vi "Configure Session.vi"(8 "error in":errorcluster, 11 "Plugin in":refnum<class "Dynamic Channel.lvclass">) -> (0 "error out":errorcluster, 3 "Plugin out":refnum<class "Dynamic Channel.lvclass">)   [LabVIEW 2020, in "Dynamic Channel.lvlib" / "Dynamic Channel.lvclass"]
uses:
  Dynamic Channel.lvclass
  C:/Program Files/National Instruments/LabVIEW 2020/vi.lib/FlexLogger/SDK/PluginSDK.lvlibp/PEFClasses/SDK/Plugin/Plugin.lvclass
  Dynamic Channel.lvclass/Dynamic Channel.ctl
  <vilib>/FlexLogger/SDK/PluginSDK.lvlibp/PEFClasses/SDK/Producer Channel/Producer Channel.lvclass
  C:/Program Files/National Instruments/LabVIEW 2020/vi.lib/FlexLogger/SDK/PluginSDK.lvlibp/PEFClasses/SDK/Channel/Channel.lvclass
  <vilib>/FlexLogger/SDK/PluginSDK.lvlibp/PEFClasses/SDK/Plugin/ParameterAccess/Read I32.vi
  <vilib>/FlexLogger/SDK/PluginSDK.lvlibp/PEFClasses/SDK/Plugin/ParameterAccess/Write I32.vi
  <vilib>/FlexLogger/SDK/PluginSDK.lvlibp/PEFClasses/SDK/Producer Channel/Create Producer Channel.vi
  <vilib>/FlexLogger/SDK/PluginSDK.lvlibp/PEFClasses/SDK/Channel/ParameterAccess/Write DBL.vi
  <vilib>/FlexLogger/SDK/PluginSDK.lvlibp/PEFClasses/SDK/Channel/ParameterAccess/Write Single Channel.vi
  <vilib>/FlexLogger/SDK/PluginSDK.lvlibp/PEFClasses/SDK/Plugin/Plugin.lvclass
  <vilib>/FlexLogger/SDK/PluginSDK.lvlibp
  <vilib>/FlexLogger/SDK/PluginSDK.lvlibp/PEFClasses/SDK/Channel/Channel.lvclass
  C:/Program Files/National Instruments/LabVIEW 2020/vi.lib/FlexLogger/SDK/PluginSDK.lvlibp/PEFClasses/SDK/Producer Channel/Producer Channel.lvclass
  C:/Program Files/National Instruments/LabVIEW 2020/vi.lib/FlexLogger/SDK/PluginSDK.lvlibp/PEFClasses/SDK/Processing Element/Processing Element.lvclass
  C:/Users/Localization Tester/Documents/LabVIEW Projects/FlexLogger IO Plugins/Dynamic Channel/Dynamic Channel.lvclass
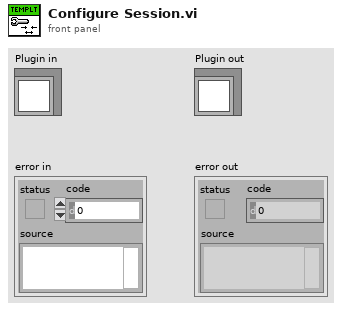
[diagram p1: front panel]
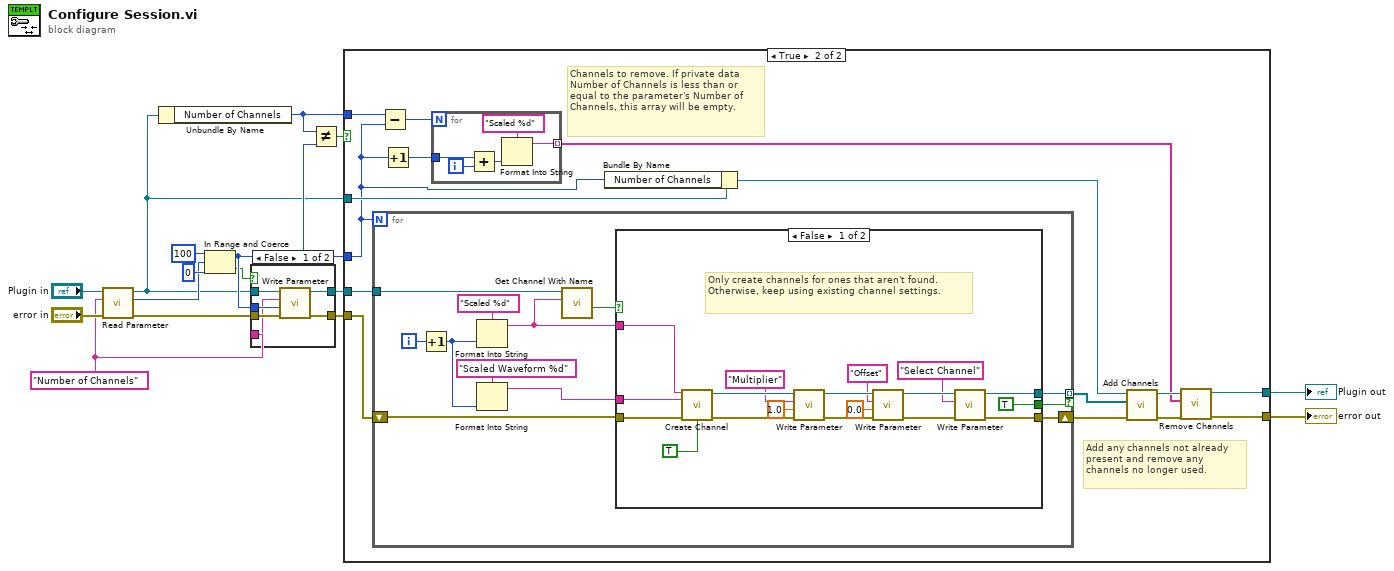
[diagram p0: block diagram]
diagram:
  w7 = "Number of Channels" ("Name (Unique Channel Identifier)")
  n1 = call-poly <vilib>:"Read Parameter.vi"("error in (no error)"="error in", "Name"=w7, "Plugin in"="Plugin in") -> ("error out"=w10:errorcluster, "Value"=w9:i32, "Plugin out"=w3:refnum<class "Dynamic Channel.lvclass">)  [unwired: 5 in, 1 out]
  n2 = Unbundle By Name(w3) -> ("Number of Channels"=w13:i32)
  n3 = In Range and Coerce(upper limit=100, x=w9, lower limit=0) -> (coerced(x)=w8:i32, In Range?=w6:bool)
  n4 = case shown="False" w6 {
    tunnel: w3 -> [w22 w24]
    tunnel: w10 -> [w21 w23]
    tunnel: w8 -> [w20 _]
    tunnel: w7 -> [w19 _]
    tunnel: [w18 w24] -> w5
    tunnel: [w17 w23] -> w4
    frame False {
      n5 = call-poly <vilib>:"Write Parameter.vi"("error in (no error)"=w21, "Value"=w20, "Name"=w19, "Plugin in"=w22) -> ("error out"=w17:errorcluster, "Plugin out"=w18:refnum<class "Dynamic Channel.lvclass">)  [unwired: 6 in]
    }
    frame True {
    }
  }
  n6 = Not Equal?(x=w13, y=w8) -> (x != y?=w14:bool)
  n7 = case shown="True" w14 {
    tunnel: w13 -> [_ w41]
    tunnel: w8 -> [_ w36]
    tunnel: w5 -> [w26 w38]
    tunnel: w4 -> [w25 w35]
    tunnel: w3 -> [_ w37]
    tunnel: [w26 w28] -> w2
    tunnel: [w25 w27] -> w1
    frame False {
    }
    frame True {
      # "Add any channels not already present and remove any channels no longer used."
      # "Channels to remove. If private data Number of Channels is less than or equal to the parameter's Number of Channels, this array will be empty."
      n8 = for {
        N: w36 -> [_]
        tunnel: w38 -> [w49]
        tunnel: [w45] -> w32 mode=indexing if=w44
        shift-right: [w43] -> w33
        shift-left: w35 -> [w42]
        i -> [w52]
        n9 = Increment(x=w52) -> (x+1=w51:i32)
        n10 = Format Into String(format string="Scaled %d", w51) -> (resulting string=w46:string)  [unwired: 2 in, 1 out]
        n11 = Format Into String(format string="Scaled Waveform %d", w51) -> (resulting string=w47:string)  [unwired: 2 in, 1 out]
        n12 = call <vilib>:"Get Channel With Name.vi"("Name"=w46, "Plugin in"=w49) -> ("Found?"=w48:bool)  [unwired: 7 in, 2 out]
        n13 = case shown="False" w48 {
          tunnel: w47 -> [w70 _]
          tunnel: w46 -> [w71 _]
          tunnel: [w58 _] -> w45
          tunnel: [TRUE _] -> w44
          tunnel: [w56 w72] -> w43
          tunnel: w42 -> [w55 w72]
          frame False {
            # "Only create channels for ones that aren't found. Otherwise, keep using existing channel settings."
            n14 = call-poly <vilib>:"Create Channel.vi"("Unique Channel Identifier"=w71, "Default Channel Name"=w70, "error in (no error)"=w55, "Can Disable?"=TRUE) -> ("Producer Channel"=w69:refnum<class "Producer Channel.lvclass">, "error out"=w66:errorcluster)  [unwired: 10 in]
            n15 = call-poly <vilib>:"Write Parameter.vi"("error in (no error)"=w66, "Value"=1.0, "Name"="Multiplier" ("Name (Unique Channel Identifier)"), "Channel in"=w69) -> ("error out"=w64:errorcluster, "Channel out"=w65:refnum<class "Producer Channel.lvclass">)  [unwired: 6 in]
            n16 = call-poly <vilib>:"Write Parameter.vi"("error in (no error)"=w64, "Value"=0.0, "Name"="Offset" ("Name (Unique Channel Identifier)"), "Channel in"=w65) -> ("error out"=w60:errorcluster, "Channel out"=w61:refnum<class "Producer Channel.lvclass">)  [unwired: 6 in]
            n17 = call-poly <vilib>:"Write Parameter.vi"("error in (no error)"=w60, "Name (Unique Channel Identifier)"="Select Channel", "Channel in"=w61) -> ("error out"=w56:errorcluster, "Channel out"=w58:refnum<class "Producer Channel.lvclass">)  [unwired: 7 in]
          }
          frame True {
          }
        }
      }
      n18 = Subtract(x=w41, y=w36) -> (x-y=w40:i32)
      n19 = Increment(x=w36) -> (x+1=w39:i32)
      n20 = for {
        N: w40 -> [_]
        tunnel: [w76] -> w29 mode=indexing
        tunnel: w39 -> [w74]
        i -> [w75]
        n21 = Add(x=w74, y=w75) -> (x+y=w73:i32)
        n22 = Format Into String(format string="Scaled %d", w73) -> (resulting string=w76:string)  [unwired: 2 in, 1 out]
      }
      n23 = Bundle By Name(cluster=w37, "Number of Channels"=w36) -> (w34:refnum<class "Dynamic Channel.lvclass">)
      n24 = call <vilib>:"Add Channels.vi"("error in (no error)"=w33, "Channels"=w32, "Plugin in"=w34) -> ("error out"=w31:errorcluster, "Plugin out"=w30:refnum<class "Dynamic Channel.lvclass">)  [unwired: 7 in]
      n25 = call-dynamic "Remove Channels.vi"("error in (no error)"=w31, "Unique Channel Identifiers to Delete"=w29, "Plugin in"=w30) -> ("error out"=w27:errorcluster, "Plugin out"=w28:refnum<class "Dynamic Channel.lvclass">)  [unwired: 7 in]
    }
  }
  "error out" <- w1
  "Plugin out" <- w2
